vi "Main.vi"(7 "sweep rate, /min":dbl=0.2, 8 "sweep to:":dbl=4.0, 9 "sweep":T8(radio)=enum."2636a_smub") -> ()   [LabVIEW 2021] (continued)
                    }
                    frame True {
                      n3679 = flat-sequence {
                        tunnel: [w4987] -> w4981
                        tunnel: [w4986] -> w4980
                        tunnel: [w4985] -> w4979
                        frame #0 {
                          n3680 = property on="HandleOut" class="Clust (strict)"() -> ("Value"=w4989:T1)  [unwired: 2 in, 2 out]
                          n3681 = call "MFLIcontrol.vi"("MFLI function"=MFLIcommand."measure XY on demod2", "handle in"=w4989) -> ("Demod Sample Out 2"=w4984:T20)  [unwired: 5 in, 4 out]
                          n3682 = Unbundle(w4984) -> ("X (Vrms)"=w4987:dbl, "Y (Vrms)"=w4986:dbl, "Freq (Hz)"=w4985:dbl)  [unwired: 6 out]
                        }
                      }
                      n3683 = Build Array (concatenate)(w4983, w4981, w4980, w4979) -> (w4982:dbl[])
                    }
                  }
                  n3684 = property on="data" class="Arr (strict)"("Value"=w4976) -> ()  [unwired: 2 in, 2 out]
                }
                frame #42 {
                  # "Measure MFLI_V if \nit is checked"
                  n3685 = property on="MFLI1_d3" class="Bool (strict)"() -> ("Value"=w4990:bool)  [unwired: 2 in, 2 out]
                  n3686 = property on="data" class="Arr (strict)"() -> ("Value"=w4992:dbl[])  [unwired: 2 in, 2 out]
                  n3687 = case shown="True" w4990 {
                    tunnel: w4992 -> [w4993 w4998]
                    tunnel: [w4993 w4997] -> w4991
                    frame False {
                      # "We are not recording Step Value if it is linetrace"
                    }
                    frame True {
                      n3688 = flat-sequence {
                        tunnel: [w5002] -> w4996
                        tunnel: [w5001] -> w4995
                        tunnel: [w5000] -> w4994
                        frame #0 {
                          n3689 = property on="HandleOut" class="Clust (strict)"() -> ("Value"=w5004:T1)  [unwired: 2 in, 2 out]
                          n3690 = call "MFLIcontrol.vi"("MFLI function"=MFLIcommand."measure XY on demod3", "handle in"=w5004) -> ("Demod Sample Out 2"=w4999:T20)  [unwired: 5 in, 4 out]
                          n3691 = Unbundle(w4999) -> ("X (Vrms)"=w5002:dbl, "Y (Vrms)"=w5001:dbl, "Freq (Hz)"=w5000:dbl)  [unwired: 6 out]
                        }
                      }
                      n3692 = Build Array (concatenate)(w4998, w4996, w4995, w4994) -> (w4997:dbl[])
                    }
                  }
                  n3693 = property on="data" class="Arr (strict)"("Value"=w4991) -> ()  [unwired: 2 in, 2 out]
                }
                frame #43 {
                  # "Measure MFLI_V if \nit is checked"
                  n3694 = property on="MFLI2_d0" class="Bool (strict)"() -> ("Value"=w5005:bool)  [unwired: 2 in, 2 out]
                  n3695 = property on="data" class="Arr (strict)"() -> ("Value"=w5007:dbl[])  [unwired: 2 in, 2 out]
                  n3696 = case shown="True" w5005 {
                    tunnel: w5007 -> [w5008 w5013]
                    tunnel: [w5008 w5012] -> w5006
                    frame False {
                      # "We are not recording Step Value if it is linetrace"
                    }
                    frame True {
                      n3697 = flat-sequence {
                        tunnel: [w5017] -> w5011
                        tunnel: [w5016] -> w5010
                        tunnel: [w5015] -> w5009
                        frame #0 {
                          n3698 = property on="HandleOut 2" class="Clust (strict)"() -> ("Value"=w5019:T21)  [unwired: 2 in, 2 out]
                          n3699 = call "MFLIcontrol.vi"("MFLI function"=MFLIcommand."measure XY on demod0", "handle in"=w5019) -> ("Demod Sample Out 2"=w5014:T20)  [unwired: 5 in, 4 out]
                          n3700 = Unbundle(w5014) -> ("X (Vrms)"=w5017:dbl, "Y (Vrms)"=w5016:dbl, "Freq (Hz)"=w5015:dbl)  [unwired: 6 out]
                        }
                      }
                      n3701 = Build Array (concatenate)(w5013, w5011, w5010, w5009) -> (w5012:dbl[])
                    }
                  }
                  n3702 = property on="data" class="Arr (strict)"("Value"=w5006) -> ()  [unwired: 2 in, 2 out]
                }
                frame #44 {
                  # "Measure MFLI_V if \nit is checked"
                  n3703 = property on="MFLI2_d1" class="Bool (strict)"() -> ("Value"=w5020:bool)  [unwired: 2 in, 2 out]
                  n3704 = property on="data" class="Arr (strict)"() -> ("Value"=w5022:dbl[])  [unwired: 2 in, 2 out]
                  n3705 = case shown="True" w5020 {
                    tunnel: w5022 -> [w5023 w5028]
                    tunnel: [w5023 w5027] -> w5021
                    frame False {
                      # "We are not recording Step Value if it is linetrace"
                    }
                    frame True {
                      n3706 = flat-sequence {
                        tunnel: [w5032] -> w5026
                        tunnel: [w5031] -> w5025
                        tunnel: [w5030] -> w5024
                        frame #0 {
                          n3707 = property on="HandleOut 2" class="Clust (strict)"() -> ("Value"=w5034:T21)  [unwired: 2 in, 2 out]
                          n3708 = call "MFLIcontrol.vi"("MFLI function"=MFLIcommand."measure XY on demod1", "handle in"=w5034) -> ("Demod Sample Out 2"=w5029:T20)  [unwired: 5 in, 4 out]
                          n3709 = Unbundle(w5029) -> ("X (Vrms)"=w5032:dbl, "Y (Vrms)"=w5031:dbl, "Freq (Hz)"=w5030:dbl)  [unwired: 6 out]
                        }
                      }
                      n3710 = Build Array (concatenate)(w5028, w5026, w5025, w5024) -> (w5027:dbl[])
                    }
                  }
                  n3711 = property on="data" class="Arr (strict)"("Value"=w5021) -> ()  [unwired: 2 in, 2 out]
                }
                frame #45 {
                  # "Measure MFLI_V if \nit is checked"
                  n3712 = property on="MFLI2_d2" class="Bool (strict)"() -> ("Value"=w5035:bool)  [unwired: 2 in, 2 out]
                  n3713 = property on="data" class="Arr (strict)"() -> ("Value"=w5037:dbl[])  [unwired: 2 in, 2 out]
                  n3714 = case shown="True" w5035 {
                    tunnel: w5037 -> [w5038 w5043]
                    tunnel: [w5038 w5042] -> w5036
                    frame False {
                      # "We are not recording Step Value if it is linetrace"
                    }
                    frame True {
                      n3715 = flat-sequence {
                        tunnel: [w5047] -> w5041
                        tunnel: [w5046] -> w5040
                        tunnel: [w5045] -> w5039
                        frame #0 {
                          n3716 = property on="HandleOut 2" class="Clust (strict)"() -> ("Value"=w5049:T21)  [unwired: 2 in, 2 out]
                          n3717 = call "MFLIcontrol.vi"("MFLI function"=MFLIcommand."measure XY on demod2", "handle in"=w5049) -> ("Demod Sample Out 2"=w5044:T20)  [unwired: 5 in, 4 out]
                          n3718 = Unbundle(w5044) -> ("X (Vrms)"=w5047:dbl, "Y (Vrms)"=w5046:dbl, "Freq (Hz)"=w5045:dbl)  [unwired: 6 out]
                        }
                      }
                      n3719 = Build Array (concatenate)(w5043, w5041, w5040, w5039) -> (w5042:dbl[])
                    }
                  }
                  n3720 = property on="data" class="Arr (strict)"("Value"=w5036) -> ()  [unwired: 2 in, 2 out]
                }
                frame #46 {
                  # "Measure MFLI_V if \nit is checked"
                  n3721 = property on="MFLI2_d3" class="Bool (strict)"() -> ("Value"=w5050:bool)  [unwired: 2 in, 2 out]
                  n3722 = property on="data" class="Arr (strict)"() -> ("Value"=w5052:dbl[])  [unwired: 2 in, 2 out]
                  n3723 = case shown="True" w5050 {
                    tunnel: w5052 -> [w5053 w5058]
                    tunnel: [w5053 w5057] -> w5051
                    frame False {
                      # "We are not recording Step Value if it is linetrace"
                    }
                    frame True {
                      n3724 = flat-sequence {
                        tunnel: [w5062] -> w5056
                        tunnel: [w5061] -> w5055
                        tunnel: [w5060] -> w5054
                        frame #0 {
                          n3725 = property on="HandleOut 2" class="Clust (strict)"() -> ("Value"=w5064:T21)  [unwired: 2 in, 2 out]
                          n3726 = call "MFLIcontrol.vi"("MFLI function"=MFLIcommand."measure XY on demod3", "handle in"=w5064) -> ("Demod Sample Out 2"=w5059:T20)  [unwired: 5 in, 4 out]
                          n3727 = Unbundle(w5059) -> ("X (Vrms)"=w5062:dbl, "Y (Vrms)"=w5061:dbl, "Freq (Hz)"=w5060:dbl)  [unwired: 6 out]
                        }
                      }
                      n3728 = Build Array (concatenate)(w5058, w5056, w5055, w5054) -> (w5057:dbl[])
                    }
                  }
                  n3729 = property on="data" class="Arr (strict)"("Value"=w5051) -> ()  [unwired: 2 in, 2 out]
                }
                frame #47 {
                  # "Measure MFLI_V if \nit is checked"
                  n3730 = property on="MFLI3_d0" class="Bool (strict)"() -> ("Value"=w5065:bool)  [unwired: 2 in, 2 out]
                  n3731 = property on="data" class="Arr (strict)"() -> ("Value"=w5067:dbl[])  [unwired: 2 in, 2 out]
                  n3732 = case shown="True" w5065 {
                    tunnel: w5067 -> [w5068 w5073]
                    tunnel: [w5068 w5072] -> w5066
                    frame False {
                      # "We are not recording Step Value if it is linetrace"
                    }
                    frame True {
                      n3733 = flat-sequence {
                        tunnel: [w5077] -> w5071
                        tunnel: [w5076] -> w5070
                        tunnel: [w5075] -> w5069
                        frame #0 {
                          n3734 = property on="HandleOut 3" class="Clust (strict)"() -> ("Value"=w5079:T1)  [unwired: 2 in, 2 out]
                          n3735 = call "MFLIcontrol.vi"("MFLI function"=MFLIcommand."measure XY on demod0", "handle in"=w5079) -> ("Demod Sample Out 2"=w5074:T20)  [unwired: 5 in, 4 out]
                          n3736 = Unbundle(w5074) -> ("X (Vrms)"=w5077:dbl, "Y (Vrms)"=w5076:dbl, "Freq (Hz)"=w5075:dbl)  [unwired: 6 out]
                        }
                      }
                      n3737 = Build Array (concatenate)(w5073, w5071, w5070, w5069) -> (w5072:dbl[])
                    }
                  }
                  n3738 = property on="data" class="Arr (strict)"("Value"=w5066) -> ()  [unwired: 2 in, 2 out]
                }
                frame #48 {
                  # "Measure MFLI_V if \nit is checked"
                  n3739 = property on="MFLI3_d1" class="Bool (strict)"() -> ("Value"=w5080:bool)  [unwired: 2 in, 2 out]
                  n3740 = property on="data" class="Arr (strict)"() -> ("Value"=w5082:dbl[])  [unwired: 2 in, 2 out]
                  n3741 = case shown="True" w5080 {
                    tunnel: w5082 -> [w5083 w5088]
                    tunnel: [w5083 w5087] -> w5081
                    frame False {
                      # "We are not recording Step Value if it is linetrace"
                    }
                    frame True {
                      n3742 = flat-sequence {
                        tunnel: [w5092] -> w5086
                        tunnel: [w5091] -> w5085
                        tunnel: [w5090] -> w5084
                        frame #0 {
                          n3743 = property on="HandleOut 3" class="Clust (strict)"() -> ("Value"=w5094:T1)  [unwired: 2 in, 2 out]
                          n3744 = call "MFLIcontrol.vi"("MFLI function"=MFLIcommand."measure XY on demod1", "handle in"=w5094) -> ("Demod Sample Out 2"=w5089:T20)  [unwired: 5 in, 4 out]
                          n3745 = Unbundle(w5089) -> ("X (Vrms)"=w5092:dbl, "Y (Vrms)"=w5091:dbl, "Freq (Hz)"=w5090:dbl)  [unwired: 6 out]
                        }
                      }
                      n3746 = Build Array (concatenate)(w5088, w5086, w5085, w5084) -> (w5087:dbl[])
                    }
                  }
                  n3747 = property on="data" class="Arr (strict)"("Value"=w5081) -> ()  [unwired: 2 in, 2 out]
                }
                frame #49 {
                  # "Measure MFLI_V if \nit is checked"
                  n3748 = property on="MFLI3_d2" class="Bool (strict)"() -> ("Value"=w5095:bool)  [unwired: 2 in, 2 out]
                  n3749 = property on="data" class="Arr (strict)"() -> ("Value"=w5097:dbl[])  [unwired: 2 in, 2 out]
                  n3750 = case shown="True" w5095 {
                    tunnel: w5097 -> [w5098 w5103]
                    tunnel: [w5098 w5102] -> w5096
                    frame False {
                      # "We are not recording Step Value if it is linetrace"
                    }
                    frame True {
                      n3751 = flat-sequence {
                        tunnel: [w5107] -> w5101
                        tunnel: [w5106] -> w5100
                        tunnel: [w5105] -> w5099
                        frame #0 {
                          n3752 = property on="HandleOut 3" class="Clust (strict)"() -> ("Value"=w5109:T1)  [unwired: 2 in, 2 out]
                          n3753 = call "MFLIcontrol.vi"("MFLI function"=MFLIcommand."measure XY on demod2", "handle in"=w5109) -> ("Demod Sample Out 2"=w5104:T20)  [unwired: 5 in, 4 out]
                          n3754 = Unbundle(w5104) -> ("X (Vrms)"=w5107:dbl, "Y (Vrms)"=w5106:dbl, "Freq (Hz)"=w5105:dbl)  [unwired: 6 out]
                        }
                      }
                      n3755 = Build Array (concatenate)(w5103, w5101, w5100, w5099) -> (w5102:dbl[])
                    }
                  }
                  n3756 = property on="data" class="Arr (strict)"("Value"=w5096) -> ()  [unwired: 2 in, 2 out]
                }
                frame #50 {
                  # "Measure MFLI_V if \nit is checked"
                  n3757 = property on="MFLI3_d3" class="Bool (strict)"() -> ("Value"=w5110:bool)  [unwired: 2 in, 2 out]
                  n3758 = property on="data" class="Arr (strict)"() -> ("Value"=w5112:dbl[])  [unwired: 2 in, 2 out]
                  n3759 = case shown="True" w5110 {
                    tunnel: w5112 -> [w5113 w5118]
                    tunnel: [w5113 w5117] -> w5111
                    frame False {
                      # "We are not recording Step Value if it is linetrace"
                    }
                    frame True {
                      n3760 = flat-sequence {
                        tunnel: [w5122] -> w5116
                        tunnel: [w5121] -> w5115
                        tunnel: [w5120] -> w5114
                        frame #0 {
                          n3761 = property on="HandleOut 3" class="Clust (strict)"() -> ("Value"=w5124:T1)  [unwired: 2 in, 2 out]
                          n3762 = call "MFLIcontrol.vi"("MFLI function"=MFLIcommand."measure XY on demod3", "handle in"=w5124) -> ("Demod Sample Out 2"=w5119:T20)  [unwired: 5 in, 4 out]
                          n3763 = Unbundle(w5119) -> ("X (Vrms)"=w5122:dbl, "Y (Vrms)"=w5121:dbl, "Freq (Hz)"=w5120:dbl)  [unwired: 6 out]
                        }
                      }
                      n3764 = Build Array (concatenate)(w5118, w5116, w5115, w5114) -> (w5117:dbl[])
                    }
                  }
                  n3765 = property on="data" class="Arr (strict)"("Value"=w5111) -> ()  [unwired: 2 in, 2 out]
                }
                frame #51 {
                  # "Measure MFLI_V if \nit is checked"
                  n3766 = property on="MFLI4_d0" class="Bool (strict)"() -> ("Value"=w5125:bool)  [unwired: 2 in, 2 out]
                  n3767 = property on="data" class="Arr (strict)"() -> ("Value"=w5127:dbl[])  [unwired: 2 in, 2 out]
                  n3768 = case shown="True" w5125 {
                    tunnel: w5127 -> [w5128 w5133]
                    tunnel: [w5128 w5132] -> w5126
                    frame False {
                      # "We are not recording Step Value if it is linetrace"
                    }
                    frame True {
                      n3769 = flat-sequence {
                        tunnel: [w5137] -> w5131
                        tunnel: [w5136] -> w5130
                        tunnel: [w5135] -> w5129
                        frame #0 {
                          n3770 = property on="HandleOut 4" class="Clust (strict)"() -> ("Value"=w5139:T21)  [unwired: 2 in, 2 out]
                          n3771 = call "MFLIcontrol.vi"("MFLI function"=MFLIcommand."measure XY on demod0", "handle in"=w5139) -> ("Demod Sample Out 2"=w5134:T20)  [unwired: 5 in, 4 out]
                          n3772 = Unbundle(w5134) -> ("X (Vrms)"=w5137:dbl, "Y (Vrms)"=w5136:dbl, "Freq (Hz)"=w5135:dbl)  [unwired: 6 out]
                        }
                      }
                      n3773 = Build Array (concatenate)(w5133, w5131, w5130, w5129) -> (w5132:dbl[])
                    }
                  }
                  n3774 = property on="data" class="Arr (strict)"("Value"=w5126) -> ()  [unwired: 2 in, 2 out]
                }
                frame #52 {
                  # "Measure MFLI_V if \nit is checked"
                  n3775 = property on="MFLI4_d1" class="Bool (strict)"() -> ("Value"=w5140:bool)  [unwired: 2 in, 2 out]
                  n3776 = property on="data" class="Arr (strict)"() -> ("Value"=w5142:dbl[])  [unwired: 2 in, 2 out]
                  n3777 = case shown="True" w5140 {
                    tunnel: w5142 -> [w5143 w5148]
                    tunnel: [w5143 w5147] -> w5141
                    frame False {
                      # "We are not recording Step Value if it is linetrace"
                    }
                    frame True {
                      n3778 = flat-sequence {
                        tunnel: [w5152] -> w5146
                        tunnel: [w5151] -> w5145
                        tunnel: [w5150] -> w5144
                        frame #0 {
                          n3779 = property on="HandleOut 4" class="Clust (strict)"() -> ("Value"=w5154:T21)  [unwired: 2 in, 2 out]
                          n3780 = call "MFLIcontrol.vi"("MFLI function"=MFLIcommand."measure XY on demod1", "handle in"=w5154) -> ("Demod Sample Out 2"=w5149:T20)  [unwired: 5 in, 4 out]
                          n3781 = Unbundle(w5149) -> ("X (Vrms)"=w5152:dbl, "Y (Vrms)"=w5151:dbl, "Freq (Hz)"=w5150:dbl)  [unwired: 6 out]
                        }
                      }
                      n3782 = Build Array (concatenate)(w5148, w5146, w5145, w5144) -> (w5147:dbl[])
                    }
                  }
                  n3783 = property on="data" class="Arr (strict)"("Value"=w5141) -> ()  [unwired: 2 in, 2 out]
                }
                frame #53 {
                  # "Measure MFLI_V if \nit is checked"
                  n3784 = property on="MFLI4_d2" class="Bool (strict)"() -> ("Value"=w5155:bool)  [unwired: 2 in, 2 out]
                  n3785 = property on="data" class="Arr (strict)"() -> ("Value"=w5157:dbl[])  [unwired: 2 in, 2 out]
                  n3786 = case shown="True" w5155 {
                    tunnel: w5157 -> [w5158 w5163]
                    tunnel: [w5158 w5162] -> w5156
                    frame False {
                      # "We are not recording Step Value if it is linetrace"
                    }
                    frame True {
                      n3787 = flat-sequence {
                        tunnel: [w5167] -> w5161
                        tunnel: [w5166] -> w5160
                        tunnel: [w5165] -> w5159
                        frame #0 {
                          n3788 = property on="HandleOut 4" class="Clust (strict)"() -> ("Value"=w5169:T21)  [unwired: 2 in, 2 out]
                          n3789 = call "MFLIcontrol.vi"("MFLI function"=MFLIcommand."measure XY on demod2", "handle in"=w5169) -> ("Demod Sample Out 2"=w5164:T20)  [unwired: 5 in, 4 out]
                          n3790 = Unbundle(w5164) -> ("X (Vrms)"=w5167:dbl, "Y (Vrms)"=w5166:dbl, "Freq (Hz)"=w5165:dbl)  [unwired: 6 out]
                        }
                      }
                      n3791 = Build Array (concatenate)(w5163, w5161, w5160, w5159) -> (w5162:dbl[])
                    }
                  }
                  n3792 = property on="data" class="Arr (strict)"("Value"=w5156) -> ()  [unwired: 2 in, 2 out]
                }
                frame #54 {
                  # "Measure MFLI_V if \nit is checked"
                  n3793 = property on="MFLI4_d3" class="Bool (strict)"() -> ("Value"=w5170:bool)  [unwired: 2 in, 2 out]
                  n3794 = property on="data" class="Arr (strict)"() -> ("Value"=w5172:dbl[])  [unwired: 2 in, 2 out]
                  n3795 = case shown="True" w5170 {
                    tunnel: w5172 -> [w5173 w5178]
                    tunnel: [w5173 w5177] -> w5171
                    frame False {
                      # "We are not recording Step Value if it is linetrace"
                    }
                    frame True {
                      n3796 = flat-sequence {
                        tunnel: [w5182] -> w5176
                        tunnel: [w5181] -> w5175
                        tunnel: [w5180] -> w5174
                        frame #0 {
                          n3797 = property on="HandleOut 4" class="Clust (strict)"() -> ("Value"=w5184:T21)  [unwired: 2 in, 2 out]
                          n3798 = call "MFLIcontrol.vi"("MFLI function"=MFLIcommand."measure XY on demod3", "handle in"=w5184) -> ("Demod Sample Out 2"=w5179:T20)  [unwired: 5 in, 4 out]
                          n3799 = Unbundle(w5179) -> ("X (Vrms)"=w5182:dbl, "Y (Vrms)"=w5181:dbl, "Freq (Hz)"=w5180:dbl)  [unwired: 6 out]
                        }
                      }
                      n3800 = Build Array (concatenate)(w5178, w5176, w5175, w5174) -> (w5177:dbl[])
                    }
                  }
                  n3801 = property on="data" class="Arr (strict)"("Value"=w5171) -> ()  [unwired: 2 in, 2 out]
                }
                frame #55 {
                  # "Measure MFLI_V if \nit is checked"
                  n3802 = property on="MFLI1_AuxOut0" class="Bool (strict)"() -> ("Value"=w5185:bool)  [unwired: 2 in, 2 out]
                  n3803 = property on="data" class="Arr (strict)"() -> ("Value"=w5187:dbl[])  [unwired: 2 in, 2 out]
                  n3804 = case shown="True" w5185 {
                    tunnel: w5187 -> [w5188 w5190]
                    tunnel: [w5188 w5191] -> w5186
                    frame False {
                      # "We are not recording Step Value if it is linetrace"
                    }
                    frame True {
                      n3805 = flat-sequence {
                        tunnel: [w5192] -> w5189
                        frame #0 {
                          n3806 = property on="HandleOut" class="Clust (strict)"() -> ("Value"=w5194:T1)  [unwired: 2 in, 2 out]
                          n3807 = call "MFLIcontrol.vi"("MFLI function"=MFLIcommand."Get AuxOut0", "handle in"=w5194) -> ("AuxOut0_Ampl"=w5192:dbl)  [unwired: 5 in, 4 out]
                        }
                      }
                      n3808 = Build Array (concatenate)(w5190, w5189) -> (w5191:dbl[])
                    }
                  }
                  n3809 = property on="data" class="Arr (strict)"("Value"=w5186) -> ()  [unwired: 2 in, 2 out]
                }
              }
            }
            frame #4 {
              n3810 = property on="data" class="Arr (strict)"() -> ("Value"=w5195:dbl[])  [unwired: 2 in, 2 out]
            }
          }
          n3811 = stacked-sequence "add data to array" {
            tunnel: w4336 -> [w4348]
            tunnel: [w4347] -> w4335
            tunnel: w4334 -> [w4346]
            frame #0 {
              n3812 = Build Array (concatenate)(w4348, w4346) -> (w4347:dbl[][])
            }
          }
          n3813 = stacked-sequence "plot selected measurements" {
            seq-local: [_ w4371 _] -> [_ _ w4416]
            seq-local: [_ w4370 _] -> [_ _ w4417]
            tunnel: w4335 -> [_ w4369 _]
            frame #0 {
              n3814 = property on="XY Graph" class="XYGraph (strict)"("ActYScl"=0 ("Active Y Scale")) -> (error out=w4354:errorcluster)  [unwired: 2 in, 1 out]
              n3815 = property on="Show cursor" class="Bool (strict)"() -> ("Value"=w4349:bool)  [unwired: 2 in, 2 out]
              n3816 = property on="Xaxis" class="Ring (strict)"() -> ("Value"=w4359:u16)  [unwired: 2 in, 2 out]
              n3817 = property on="Yaxis" class="Ring (strict)"(error in=w4354) -> (error out=w4353:errorcluster, "RingText.Text"=w4352:string)  [unwired: 1 in, 1 out]
              n3818 = property on="XY Graph" class="XYGraph (strict)"("Cursor.Visible"=w4349) -> ()  [unwired: 2 in, 2 out]
              n3819 = property on="Figure_axis" class="Arr (strict)"() -> ("Value"=w4360:string[])  [unwired: 2 in, 2 out]
              n3820 = property on="XY Graph" class="XYGraph (strict)"(error in=w4353, "YScale.NameLbl.Text"=w4352) -> (error out=w4350:errorcluster)  [unwired: 1 in, 1 out]
              n3821 = property on="XY Graph" class="XYGraph (strict)"(error in=w4350, "ActYScl"=1 ("Active Y Scale")) -> (error out=w4356:errorcluster)  [unwired: 1 in, 1 out]
              n3822 = property on="Yright" class="Ring (strict)"(error in=w4356) -> (error out=w4357:errorcluster, "RingText.Text"=w4351:string)  [unwired: 1 in, 1 out]
              n3823 = Index Array(array=w4360, index=w4359) -> (element=w4361:string)
              n3824 = property on="XY Graph" class="XYGraph (strict)"("XScale.NameLbl.Text"=w4361) -> ()  [unwired: 2 in, 2 out]
              n3825 = property on="XY Graph" class="XYGraph (strict)"(error in=w4357, "YScale.NameLbl.Text"=w4351) -> ()  [unwired: 1 in, 2 out]
            }
            frame #1 {
              n3826 = local read "Xaxis"() -> (w4374:u16)
              n3827 = property on="Yright" class="Ring (strict)"() -> ("Value"=w4368:u16)  [unwired: 2 in, 2 out]
              n3828 = property on="Yright" class="Ring (strict)"() -> ("RingText.Text"=w4367:string)  [unwired: 2 in, 2 out]
              n3829 = property on="Xaxis" class="Ring (strict)"() -> ("RingText.Text"=w4373:string)  [unwired: 2 in, 2 out]
              n3830 = property on="Yaxis" class="Ring (strict)"() -> ("RingText.Text"=w4372:string)  [unwired: 2 in, 2 out]
              n3831 = local read "Yaxis"() -> (w4375:u16)
              n3832 = case shown="\"formula\"" w4367 {
                tunnel: [w4380 w4387] -> w4365
                tunnel: w4368 -> [_ w4386]
                tunnel: w4369 -> [w4381 w4385]
                tunnel: [w4379 errorcluster {"status"=FALSE, "code"=0, "source"=""} ("error out")] -> _
                frame "formula" {
                  n3833 = local read "formula_variables"() -> (w4382:string[])
                  n3834 = Transpose 2D Array(2D array=w4381) -> (transposed array=w4383:dbl[][])
                  n3835 = property on="Y_right_formula" class="Str"() -> ("Value"=w4378:string)  [unwired: 2 in, 2 out]
                  n3836 = call <vilib>:"Eval Multi-Variable Array.vi"("Variables"=w4382, "X Values"=w4383, "formula"=w4378) -> ("error out"=w4379:errorcluster, "Y Values"=w4380:dbl[])  [unwired: 1 in]
                }
                frame "0", Default {
                  n3837 = Index Array(array=w4385, index (col)=w4386) -> (element=w4387:dbl[])  [unwired: 1 in]
                }
              }
              n3838 = case shown="\"formula\"" w4373 {
                tunnel: [w4398 w4403] -> w4377
                tunnel: w4374 -> [w4401 _]
                tunnel: w4369 -> [w4400 w4407]
                tunnel: [errorcluster {"status"=FALSE, "code"=0, "source"=""} ("error out") w4404] -> w4371
                tunnel: [w4398 w4403] -> w4366
                frame "0", Default {
                  n3839 = Index Array(array=w4400, index (col)=w4401) -> (element=w4398:dbl[])  [unwired: 1 in]
                }
                frame "formula" {
                  n3840 = local read "formula_variables"() -> (w4406:string[])
                  n3841 = Transpose 2D Array(2D array=w4407) -> (transposed array=w4405:dbl[][])
                  n3842 = property on="X_axis_formula" class="Str"() -> ("Value"=w4402:string)  [unwired: 2 in, 2 out]
                  n3843 = call <vilib>:"Eval Multi-Variable Array.vi"("Variables"=w4406, "X Values"=w4405, "formula"=w4402) -> ("error out"=w4404:errorcluster, "Y Values"=w4403:dbl[])  [unwired: 1 in]
                }
              }
              n3844 = case shown="\"formula\"" w4372 {
                tunnel: [w4390 w4397] -> w4376
                tunnel: w4375 -> [_ w4396]
                tunnel: w4369 -> [w4391 w4395]
                tunnel: [w4389 errorcluster {"status"=FALSE, "code"=0, "source"=""} ("error out")] -> w4370
                frame "formula" {
                  n3845 = local read "formula_variables"() -> (w4392:string[])
                  n3846 = Transpose 2D Array(2D array=w4391) -> (transposed array=w4393:dbl[][])
                  n3847 = property on="Y_left_formula" class="Str"() -> ("Value"=w4388:string)  [unwired: 2 in, 2 out]
                  n3848 = call <vilib>:"Eval Multi-Variable Array.vi"("Variables"=w4392, "X Values"=w4393, "formula"=w4388) -> ("error out"=w4389:errorcluster, "Y Values"=w4390:dbl[])  [unwired: 1 in]
                }
                frame "0", Default {
                  n3849 = Index Array(array=w4395, index (col)=w4396) -> (element=w4397:dbl[])  [unwired: 1 in]
                }
              }
              n3850 = Bundle("Y Values"=w4377, "Y Values"=w4376) -> (w4364:cluster{"Y Values":dbl[], "Y Values":dbl[]})  [unwired: 1 in]
              n3851 = Bundle("Y Values"=w4366, "Y Values"=w4365) -> (w4363:cluster{"Y Values":dbl[], "Y Values":dbl[]})  [unwired: 1 in]
              n3852 = Build Array(w4364, w4363) -> (w4362:cluster{"Y Values":dbl[], "Y Values":dbl[]}[])
              n3853 = property on="XY Graph" class="XYGraph (strict)"("Value"=w4362) -> ()  [unwired: 2 in, 2 out]
            }
            frame #2 {
              # "show if formula \nis wrong"
              n3854 = property on="Yaxis" class="Ring (strict)"() -> ("RingText.Text"=w4413:string)  [unwired: 2 in, 2 out]
              n3855 = property on="XY Graph" class="XYGraph (strict)"("Active Plot"=u32 0, "Plot.Plot Name"=w4413) -> (error out=w4414:errorcluster)  [unwired: 2 in, 1 out]
              n3856 = property on="Yright" class="Ring (strict)"() -> ("RingText.Text"=w4411:string)  [unwired: 2 in, 2 out]
              n3857 = property on="XY Graph" class="XYGraph (strict)"(error in=w4414, "Active Plot"=u32 1, "Plot.Plot Name"=w4411) -> ()  [unwired: 1 in, 2 out]
              n3858 = Unbundle By Name(w4417) -> ("status"=w4410:bool)
              n3859 = Unbundle By Name(w4416) -> ("status"=w4409:bool)
              n3860 = Unbundle By Name(w4416) -> ("status"=w4408:bool)
              n3861 = property on="status 3" class="Bool (strict)"("Value"=w4408) -> ()  [unwired: 2 in, 2 out]
              n3862 = property on="status 2" class="Bool (strict)"("Value"=w4410) -> ()  [unwired: 2 in, 2 out]
              n3863 = property on="status" class="Bool (strict)"("Value"=w4409) -> ()  [unwired: 2 in, 2 out]
            }
          }
          n3864 = stacked-sequence "set next value in the sweep" {
            tunnel: w4345 -> [w5201 _]
            tunnel: [w5201 _] -> w4344
            tunnel: w4342 -> [_ w5317]
            tunnel: w4340 -> [w5204 _]
            frame #0 {
              n3865 = local read "sweep"() -> (w5207:T8)
              n3866 = property on="Sweep Channel" class="DigNum (strict)"("Value"=w5201) -> ()  [unwired: 2 in, 2 out]
              n3867 = property on="sweep value" class="DigNum (strict)"("Value"=w5201) -> ()  [unwired: 2 in, 2 out]
              n3868 = case shown="\"AuxOut0\"" w5207 {
                tunnel: w5201 -> [w5220 w5228 w5234 w5243 w5265 _ w5267 w5290 w5308 w5311]
                tunnel: w5204 -> [_ _ _ w5242 _ _ _ _ _ _]
                frame "2400_1" {
                  # "sweep voltage on 2400 1"
                  n3869 = local read "2400 1 addr"() -> (w5222:u8)
                  n3870 = Number To Fractional String(number=w5220) -> (F-format string=w5226:string)  [unwired: 3 in]
                  n3871 = Concatenate Strings(":INIT:IMM; :SOUR:VOLT:LEV:IMM:AMPL " ("data"), w5226) -> (w5224:string)
                  n3872 = Number To Decimal String(number=w5222) -> (decimal integer string=w5221:string)  [unwired: 1 in]
                  n3873 = GPIB Write(0:w5221, 1:w5224, 2:i16 1 ("mode (0)")) -> ()  [unwired: 2 in, 2 out]
                }
                frame "2400_2" {
                  # "sweep curr on 2400 2"
                  n3874 = Number To Fractional String(number=w5228) -> (F-format string=w5233:string)  [unwired: 3 in]
                  n3875 = local read "2400 2 addr"() -> (w5230:u8)
                  n3876 = Concatenate Strings(":INIT:IMM; :SOUR:CURR:LEV:IMM:AMPL " ("data"), w5233) -> (w5231:string)
                  n3877 = Number To Decimal String(number=w5230) -> (decimal integer string=w5229:string)  [unwired: 1 in]
                  n3878 = GPIB Write(0:w5229, 1:w5231, 2:i16 1 ("mode (0)")) -> ()  [unwired: 2 in, 2 out]
                }
                frame "2400_3" {
                  # "sweep voltage on 2400 3"
                  n3879 = local read "2400 3 addr"() -> (w5236:u8)
                  n3880 = Number To Fractional String(number=w5234) -> (F-format string=w5240:string)  [unwired: 3 in]
                  n3881 = Concatenate Strings(":INIT:IMM; :SOUR:VOLT:LEV:IMM:AMPL " ("data"), w5240) -> (w5238:string)
                  n3882 = Number To Decimal String(number=w5236) -> (decimal integer string=w5235:string)  [unwired: 1 in]
                  n3883 = GPIB Write(0:w5235, 1:w5238, 2:i16 1 ("mode (0)")) -> ()  [unwired: 2 in, 2 out]
                }
                frame "2636a_smua" {
                  n3884 = property on="sweep" class="Bool (strict)"() -> ("Value"=w5241:bool)  [unwired: 2 in, 2 out]
                  n3885 = case shown="False" w5241 {
                    tunnel: w5243 -> [w5248 w5261]
                    tunnel: w5242 -> [w5245 _]
                    frame True {
                      w5246 = 30.0 ("y")
                      n3886 = Subtract(x=w5248, y=w5245) -> (x-y=w5247:dbl)
                      n3887 = Divide(x=w5247, y=w5246) -> (x/y=w5244:dbl)
                      n3888 = for {
                        N: w5246 -> [_]
                        tunnel: w5245 -> [w5254]
                        tunnel: w5244 -> [w5252]
                        i -> [w5253]
                        n3889 = Multiply(x=w5252, y=w5253) -> (x*y=w5251:dbl)
                        n3890 = local read "2614A addr"() -> (w5256:refnum<visa-resource-name>)
                        n3891 = Add(x=w5251, y=w5254) -> (x+y=w5250:dbl)
                        n3892 = call "setLevel.vi"("VISA resource name 2"=w5256, "Source"=Source."Voltage", "Channel"=Channel."a", "SourceLevel"=w5250) -> ()  [unwired: 1 in, 3 out]
                        n3893 = Wait (ms)(milliseconds to wait=u32 12) -> ()  [unwired: 1 out]
                      }
                    }
                    frame False {
                      # "sweep voltage on 2636a smua"
                      n3894 = local read "2614A addr"() -> (w5259:refnum<visa-resource-name>)
                      n3895 = call "setLevel.vi"("VISA resource name 2"=w5259, "Source"=Source."Voltage", "Channel"=Channel."a", "SourceLevel"=w5261) -> ()  [unwired: 1 in, 3 out]
                    }
                  }
                }
                frame "2636a_smub" {
                  # "sweep voltage on 2636b smua"
                  n3896 = local read "2614A addr"() -> (w5262:refnum<visa-resource-name>)
                  n3897 = call "setLevel.vi"("VISA resource name 2"=w5262, "Source"=Source."Voltage", "Channel"=Channel."b", "SourceLevel"=w5265) -> ()  [unwired: 1 in, 3 out]
                }
                frame "time_sweep", Default {
                  # "do not sweep, just time"
                }
                frame "iPS" {
                  n3898 = property on="Sweep B" class="Bool (strict)"() -> ("Value"=w5266:bool)  [unwired: 2 in, 2 out]
                  n3899 = case shown="True" w5266 {
                    tunnel: w5267 -> [_ w5268]
                    frame False {
                    }
                    frame True {
                      n3900 = stacked-sequence {
                        tunnel: w5268 -> [w5269 _ w5279 w5281]
                        frame #0 {
                          n3901 = local read "iPS_addr_sweep"() -> (w5271:refnum<visa-resource-name>)
                          n3902 = call "iPSset.vi"("Target Field, T"=w5269, "iPSSetCtrl"=iPSsetCtrl."Set Target Field", "VISA resource name"=w5271) -> ()  [unwired: 5 in, 4 out]
                        }
                        frame #1 {
                          n3903 = local read "iPS_addr_sweep"() -> (w5274:refnum<visa-resource-name>)
                          n3904 = call "iPSset.vi"("Field Rate, T/min"=0.15, "iPSSetCtrl"=iPSsetCtrl."Set Target Field Rate", "VISA resource name"=w5274) -> ()  [unwired: 5 in, 4 out]
                        }
                        frame #2 {
                          n3905 = Not Equal To 0?(x=w5279) -> (x != 0?=w5277:bool)
                          n3906 = local read "iPS_addr_sweep"() -> (w5280:refnum<visa-resource-name>)
                          n3907 = Select(t=iPSsetCtrl."Go to Field" ("iPSSetCtrl"), s=w5277, f=iPSsetCtrl."Go to Field" ("iPSSetCtrl")) -> (s? t:f=w5275:T16)
                          n3908 = call "iPSset.vi"("iPSSetCtrl"=w5275, "VISA resource name"=w5280) -> ()  [unwired: 6 in, 4 out]
                        }
                        frame #3 {
                          n3909 = while {
                            tunnel: w5281 -> [w5283]
                            stop <- w5287 stop-if-true
                            n3910 = property on="iPS _addr_step" class="VISAName"() -> ("Value"=w5286:refnum<visa-resource-name>)  [unwired: 2 in, 2 out]
                            n3911 = call "iPSread.vi"("iPSreadCtrl"=iPSreadCtrl."MagnetField", "VISA resource name"=w5286) -> ("number"=w5285:dbl)  [unwired: 6 in, 3 out]
                            n3912 = Subtract(x=w5285, y=w5283) -> (x-y=w5289:dbl)
                            n3913 = property on="Tolerance_Sweep" class="DigNum (strict)"() -> ("Value"=w5284:dbl)  [unwired: 2 in, 2 out]
                            n3914 = Absolute Value(x=w5289) -> (abs(x)=w5288:dbl)
                            n3915 = Less Or Equal?(x=w5288, y=w5284) -> (x <= y?=w5287:bool)
                          }
                        }
                      }
                    }
                  }
                }
                frame "iTC" {
                  n3916 = stacked-sequence {
                    tunnel: w5290 -> [w5292 w5297 w5300]
                    frame #0 {
                      n3917 = Decrement(x=w5292) -> (x-1=w5293:dbl)
                      n3918 = Less Or Equal To 0?(x=w5293) -> (x <= 0?=w5295:bool)
                      n3919 = Select(t=0.0, s=w5295, f=w5293) -> (s? t:f=w5291:dbl)
                      n3920 = call "TRITON_Set Temperature.vi"("setpoint"=w5291) -> ()  [unwired: 2 in, 1 out]
                    }
                    frame #1 {
                      n3921 = Less Or Equal To 0?(x=w5297) -> (x <= 0?=w5299:bool)
                      n3922 = Select(t=0.0, s=w5299, f=w5297) -> (s? t:f=w5296:dbl)
                      n3923 = call "TRITON_Set Temperature.vi"("setpoint"=w5296) -> ()  [unwired: 2 in, 1 out]
                    }
                    frame #2 {
                      n3924 = while {
                        tunnel: w5300 -> [w5304]
                        stop <- w5305 stop-if-true
                        n3925 = call "TRITON_Read Temperature.vi"("Channel"="T_Channel_sweep") -> ("Measuremet"=w5302:dbl)  [unwired: 1 in, 1 out]
                        n3926 = Subtract(x=w5302, y=w5304) -> (x-y=w5307:dbl)
                        n3927 = property on="Tolerance_Sweep" class="DigNum (strict)"() -> ("Value"=w5303:dbl)  [unwired: 2 in, 2 out]
                        n3928 = Absolute Value(x=w5307) -> (abs(x)=w5306:dbl)
                        n3929 = Less?(x=w5306, y=w5303) -> (x < y?=w5305:bool)
                      }
                    }
                  }
                }
                frame "2461" {
                  w5309 = u16 1 items=["Volts", "Current"] ("Function (0: Volts)")
                  n3930 = property on="2461_addr_sweep" class="VISAName"() -> ("Value"=w5310:refnum<visa-resource-name>)  [unwired: 2 in, 2 out]
                  n3931 = call <instrlib>:"Configure Source Level.vi"("Source Level (1.0)"=w5308, "Function (0: Volts)"=w5309, "VISA resource name"=w5310) -> ()  [unwired: 7 in, 2 out]
                }
                frame "AuxOut0" {
                  n3932 = property on="HandleOut" class="Clust (strict)"() -> ("Value"=w5313:T1)  [unwired: 2 in, 2 out]
                  n3933 = call "MFLIcontrol.vi"("Value"=w5311, "MFLI function"=MFLIcommand."Set AuxOut0", "handle in"=w5313) -> ()  [unwired: 4 in, 5 out]
                }
              }
              n3934 = property on="Offset" class="DigNum (strict)"() -> ("Value"=w5203:dbl)  [unwired: 2 in, 2 out]
              n3935 = property on="Slope" class="DigNum (strict)"() -> ("Value"=w5202:dbl)  [unwired: 2 in, 2 out]
              n3936 = Multiply(x=w5202, y=w5201) -> (x*y=w5205:dbl)
              n3937 = local read "sweep"() -> (w5200:T8)
              n3938 = property on="Lead Chanl" class="Enum (strict)"() -> ("Value"=w5199:T2)  [unwired: 2 in, 2 out]
              n3939 = property on="Double Sweep" class="Bool (strict)"() -> ("Value"=w5197:bool)  [unwired: 2 in, 2 out]
              n3940 = Add(x=w5203, y=w5205) -> (x+y=w5206:dbl)
              n3941 = Equal?(x=w5200, y=w5199) -> (x = y?=w5198:bool)
              n3942 = And(x=w5197, y=w5198) -> (x .and. y?=w5196:bool)
              n3943 = case shown="True" w5196 {
                tunnel: w5206 -> [_ w5208]
                frame False {
                }
                frame True {
                  n3944 = disable-structure shown="Enabled" {
                    disable-tunnel: w5208 -> [w5209 w5217]
                    frame Disabled {
                      # "sweep voltage on 2400 2"
                      n3945 = local read "2400 2 addr"() -> (w5210:u8)
                      n3946 = Number To Fractional String(number=w5209) -> (F-format string=w5211:string)  [unwired: 3 in]
                      n3947 = Concatenate Strings(":INIT:IMM; :SOUR:VOLT:LEV:IMM:AMPL " ("data"), w5211) -> (w5213:string)
                      n3948 = Number To Decimal String(number=w5210) -> (decimal integer string=w5214:string)  [unwired: 1 in]
                      n3949 = GPIB Write(0:w5214, 1:w5213, 2:i16 1 ("mode (0)")) -> ()  [unwired: 2 in, 2 out]
                    }
                    frame Enabled {
                      n3950 = property on="Slave Channel" class="Enum (strict)"() -> ("Value"=w5216:T3)  [unwired: 2 in, 2 out]
                      n3951 = local read "2614A addr"() -> (w5219:refnum<visa-resource-name>)
                      n3952 = call "setLevel.vi"("VISA resource name 2"=w5219, "Source"=Source."Voltage", "Channel"=w5216, "SourceLevel"=w5217) -> ()  [unwired: 1 in, 3 out]
                    }
                  }
                }
              }
            }
            frame #1 {
              # "calculate deliberate time delay for the next step"
              n3953 = Tick Count (ms)() -> (millisecond timer value=w5319:u32)
              n3954 = Subtract(x=w5319, y=w5317) -> (x-y=w5318:u32)
              n3955 = property on="time/point, sec" class="DigNum (strict)"() -> ("Value"=w5314:dbl)  [unwired: 2 in, 2 out]
              n3956 = Multiply(x=w5314, y=1000.0) -> (x*y=w5316:dbl)
              n3957 = Subtract(x=w5316, y=w5318) -> (x-y=w5315:dbl)
              n3958 = property on="time delay, ms" class="DigNum (strict)"("Value"=w5315) -> ()  [unwired: 2 in, 2 out]
            }
          }
          n3959 = Or(x=w4338, y="Stop Ramp") -> (x .or. y?=w4339:bool)
        }
        n3960 = stacked-sequence {
          tunnel: w3555 -> [_ _]
          tunnel: w3554 -> [_ w4324]
          frame #0 {
            n3961 = stacked-sequence {
              frame #0 {
                n3962 = local read "sweep"() -> (w4290:T8)
                n3963 = Equal?(x=w4290, y=T17."Radio Selection 7" ("sweep")) -> (x = y?=w4289:bool)
                n3964 = case shown="True" w4289 {
                  frame False {
                  }
                  frame True {
                    n3965 = local read "iPS_addr_sweep"() -> (w4291:refnum<visa-resource-name>)
                    n3966 = call "iPSset.vi"("iPSSetCtrl"=iPSsetCtrl."Hold", "VISA resource name"=w4291) -> ()  [unwired: 6 in, 4 out]
                  }
                }
              }
              frame #1 {
                n3967 = stacked-sequence {
                  frame #0 {
                    n3968 = property on="MFLI1_d0" class="Bool (strict)"() -> ("Value"=w4306:bool)  [unwired: 2 in, 2 out]
                    n3969 = property on="MFLI1_AuxOut0" class="Bool (strict)"() -> ("Value"=w4310:bool)  [unwired: 2 in, 2 out]
                    n3970 = property on="MFLI1_d1" class="Bool (strict)"() -> ("Value"=w4305:bool)  [unwired: 2 in, 2 out]
                    n3971 = property on="MFLI1_d2" class="Bool (strict)"() -> ("Value"=w4304:bool)  [unwired: 2 in, 2 out]
                    n3972 = property on="MFLI1_d3" class="Bool (strict)"() -> ("Value"=w4303:bool)  [unwired: 2 in, 2 out]
                    n3973 = Boolean To (0,1)(Boolean=w4305) -> (0, 1=w4301:i16)
                    n3974 = Boolean To (0,1)(Boolean=w4306) -> (0, 1=w4302:i16)
                    n3975 = Boolean To (0,1)(Boolean=w4310) -> (0, 1=w4307:i16)
                    n3976 = Boolean To (0,1)(Boolean=w4304) -> (0, 1=w4300:i16)
                    n3977 = Boolean To (0,1)(Boolean=w4303) -> (0, 1=w4299:i16)
                    n3978 = Compound Arithmetic op=ADD(w4307, w4302, w4301, w4300, w4299) -> (w4308:i16)
                    n3979 = Greater Than 0?(x=w4308) -> (x > 0?=w4309:bool)
                    n3980 = case shown="True" w4309 {
                      frame False {
                      }
                      frame True {
                        n3981 = property on="HandleOut" class="Clust (strict)"() -> ("Value"=w4311:T1)  [unwired: 2 in, 2 out]
                        n3982 = call <instrlib>:"ziClose.vi"("Handle In"=w4311) -> ()  [unwired: 3 in, 2 out]
                      }
                    }
                  }
                  frame #1 {
                    n3983 = property on="MFLI2_d0" class="Bool (strict)"() -> ("Value"=w4321:bool)  [unwired: 2 in, 2 out]
                    n3984 = property on="MFLI2_d1" class="Bool (strict)"() -> ("Value"=w4317:bool)  [unwired: 2 in, 2 out]
                    n3985 = property on="MFLI2_d2" class="Bool (strict)"() -> ("Value"=w4316:bool)  [unwired: 2 in, 2 out]
                    n3986 = property on="MFLI2_d3" class="Bool (strict)"() -> ("Value"=w4315:bool)  [unwired: 2 in, 2 out]
                    n3987 = Boolean To (0,1)(Boolean=w4316) -> (0, 1=w4312:i16)
                    n3988 = Boolean To (0,1)(Boolean=w4317) -> (0, 1=w4314:i16)
                    n3989 = Boolean To (0,1)(Boolean=w4321) -> (0, 1=w4318:i16)
                    n3990 = Boolean To (0,1)(Boolean=w4315) -> (0, 1=w4313:i16)
                    n3991 = Compound Arithmetic op=ADD(w4318, w4314, w4313, w4312) -> (w4319:i16)
                    n3992 = Greater Than 0?(x=w4319) -> (x > 0?=w4320:bool)
                    n3993 = case shown="True" w4320 {
                      frame False {
                      }
                      frame True {
                        n3994 = property on="HandleOut 2" class="Clust (strict)"() -> ("Value"=w4322:T1)  [unwired: 2 in, 2 out]
                        n3995 = call <instrlib>:"ziClose.vi"("Handle In"=w4322) -> ()  [unwired: 3 in, 2 out]
                      }
                    }
                  }
                }
                n3996 = local read "2636A smua meas v"() -> (w4298:bool)
                n3997 = local read "2636A smub meas v"() -> (w4296:bool)
                n3998 = local read "2636A smub meas i"() -> (w4295:bool)
                n3999 = local read "2636A smua meas i"() -> (w4297:bool)
                n4000 = Compound Arithmetic op=OR(w4298, w4297, w4296, w4295) -> (w4294:bool)
                n4001 = property on="Stop Ramp" class="Bool"("DisabledEnum"=T10."Disabled and Grayed Out" ("Disabled")) -> ()  [unwired: 2 in, 2 out]
                n4002 = case shown="True" w4294 {
                  frame False {
                  }
                  frame True {
                    # "close session on 2636A"
                    n4003 = local read "2614A addr"() -> (w4323:refnum<visa-resource-name>)
                    n4004 = VISA Close(VISA resource name=w4323) -> ()  [unwired: 1 in, 1 out]
                  }
                }
              }
            }
          }
          frame #1 {
            n4005 = property on="Linetrace or Mapping?" class="Bool (strict)"() -> ("Value"=w4325:bool)  [unwired: 2 in, 2 out]
            n4006 = case shown="True" w4325 {
              tunnel: w4324 -> [w4329 w4330]
              frame False {
                w4327 = T10."Enabled" ("Disabled")
                n4007 = Enqueue Element(queue=w4329, element="Idle") -> ()  [unwired: 2 in, 3 out]
                n4008 = property on="sweep" class="RadioBtnsControl (strict)"("DisabledEnum"=w4327) -> ()  [unwired: 2 in, 2 out]
                n4009 = property on="2182A 1 addr" class="DigNum (strict)"("DisabledEnum"=w4327) -> ()  [unwired: 2 in, 2 out]
                n4010 = property on="2182A 2 addr" class="DigNum (strict)"("DisabledEnum"=w4327) -> ()  [unwired: 2 in, 2 out]
                n4011 = property on="2182A 3 addr" class="DigNum (strict)"("DisabledEnum"=w4327) -> ()  [unwired: 2 in, 2 out]
                n4012 = property on="2182A 4 addr" class="DigNum (strict)"("DisabledEnum"=w4327) -> ()  [unwired: 2 in, 2 out]
                n4013 = property on="2400 1 addr" class="DigNum (strict)"("DisabledEnum"=w4327) -> ()  [unwired: 2 in, 2 out]
                n4014 = property on="Sweep Down" class="Bool"("DisabledEnum"=w4327) -> ()  [unwired: 2 in, 2 out]
                n4015 = property on="2400 2 addr" class="DigNum (strict)"("DisabledEnum"=w4327) -> ()  [unwired: 2 in, 2 out]
                n4016 = property on="2400 3 addr" class="DigNum (strict)"("DisabledEnum"=w4327) -> ()  [unwired: 2 in, 2 out]
                n4017 = property on="2614A addr" class="VISAName"("DisabledEnum"=w4327) -> ()  [unwired: 2 in, 2 out]
                n4018 = property on="SR830 1 addr" class="DigNum (strict)"("DisabledEnum"=w4327) -> ()  [unwired: 2 in, 2 out]
                n4019 = property on="SR830 2 addr" class="DigNum (strict)"("DisabledEnum"=w4327) -> ()  [unwired: 2 in, 2 out]
                n4020 = property on="SR830 3 addr" class="DigNum (strict)"("DisabledEnum"=w4327) -> ()  [unwired: 2 in, 2 out]
                n4021 = property on="SR830 4 addr" class="DigNum (strict)"("DisabledEnum"=w4327) -> ()  [unwired: 2 in, 2 out]
                n4022 = property on="Stop Ramp" class="Bool"("DisabledEnum"=T10."Disabled and Grayed Out" ("Disabled")) -> ()  [unwired: 2 in, 2 out]
              }
              frame True {
                n4023 = stacked-sequence {
                  tunnel: w4330 -> [_ w4333]
                  frame #0 {
                    n4024 = property on="Sweep Direction" class="Str"("Value"="Sweep Down" ("Sweep Direction")) -> ()  [unwired: 2 in, 2 out]
                  }
                  frame #1 {
                    n4025 = Enqueue Element(queue=w4333, element="Step to Next Value") -> ()  [unwired: 2 in, 3 out]
                  }
                }
              }
            }
          }
        }
      }
      frame "Step to Next Value" {
        n4026 = property on="Table Index" class="DigNum (strict)"() -> ("Value"=w5335:dbl)  [unwired: 2 in, 2 out]
        n4027 = property on="Step values" class="Tbl (strict)"() -> ("Value"=w5334:string[][])  [unwired: 2 in, 2 out]
        n4028 = Equal?(x=w5335, y=0) -> (x = y?=w5331:bool)
        n4029 = case shown="True" w5331 {
          tunnel: w5335 -> [w5336 w5360]
          tunnel: cluster{"Row":i32, "Column":i32} {"Row"=0, "Column"=0} ("Active Cell:Active Cell") -> [w5340 w5363]
          frame False {
            w5343 = 0 ("Column")
            n4030 = property on="Change Sweep Range" class="Bool (strict)"() -> ("Value"=w5337:bool)  [unwired: 2 in, 2 out]
            n4031 = Decrement(x=w5336) -> (x-1=w5344:dbl)
            n4032 = Bundle By Name(cluster=w5340, "Row"=w5336, "Column"=w5343) -> (w5339:cluster{"Row":i32, "Column":i32})
            n4033 = case shown="True" w5337 {
              tunnel: w5336 -> [_ w5346]
              frame False {
              }
              frame True {
                w5347 = 1 ("Column")
                w5359 = 0 ("Column")
                n4034 = Decrement(x=w5346) -> (x-1=w5358:dbl)
                n4035 = Bundle By Name(cluster=cluster{"Row":i32, "Column":i32} {"Row"=0, "Column"=0} ("Active Cell:Active Cell"), "Row"=w5346, "Column"=w5359) -> (w5356:cluster{"Row":i32, "Column":i32})
                n4036 = Decrement(x=w5346) -> (x-1=w5348:dbl)
                n4037 = Bundle By Name(cluster=w5356, "Row"=w5358, "Column"=w5359) -> (w5355:cluster{"Row":i32, "Column":i32})
                n4038 = Bundle By Name(cluster=cluster{"Row":i32, "Column":i32} {"Row"=0, "Column"=0} ("Active Cell:Active Cell"), "Row"=w5346, "Column"=w5347) -> (w5349:cluster{"Row":i32, "Column":i32})
                n4039 = Bundle By Name(cluster=w5349, "Row"=w5348, "Column"=w5347) -> (w5350:cluster{"Row":i32, "Column":i32})
                n4040 = property on="Down          Up" class="Tbl (strict)"("Active Cell"=w5355, "Cell BG Color"=u32 16711680 ("Active Cell:Cell Background Color")) -> ()  [unwired: 2 in, 2 out]
                n4041 = property on="Down          Up" class="Tbl (strict)"("Active Cell"=w5356, "Cell BG Color"=u32 16776072 ("Active Cell:Cell Background Color")) -> ()  [unwired: 2 in, 2 out]
                n4042 = property on="Down          Up" class="Tbl (strict)"("Active Cell"=w5350, "Cell BG Color"=u32 16711680 ("Active Cell:Cell Background Color")) -> ()  [unwired: 2 in, 2 out]
                n4043 = property on="Down          Up" class="Tbl (strict)"("Active Cell"=w5349, "Cell BG Color"=u32 16776072 ("Active Cell:Cell Background Color")) -> ()  [unwired: 2 in, 2 out]
              }
            }
            n4044 = Bundle By Name(cluster=w5339, "Row"=w5344, "Column"=w5343) -> (w5338:cluster{"Row":i32, "Column":i32})
            n4045 = property on="Step values" class="Tbl (strict)"("Active Cell"=w5339, "Cell BG Color"=u32 16776072 ("Active Cell:Cell Background Color")) -> ()  [unwired: 2 in, 2 out]
            n4046 = property on="Step values" class="Tbl (strict)"("Active Cell"=w5338, "Cell BG Color"=u32 16711680 ("Active Cell:Cell Background Color")) -> ()  [unwired: 2 in, 2 out]
          }
          frame True {
            n4047 = property on="Change Sweep Range" class="Bool (strict)"() -> ("Value"=w5361:bool)  [unwired: 2 in, 2 out]
            n4048 = Bundle By Name(cluster=w5363, "Row"=w5360, "Column"=0) -> (w5362:cluster{"Row":i32, "Column":i32})
            n4049 = case shown="True" w5361 {
              tunnel: w5360 -> [_ w5371]
              frame False {
              }
              frame True {
                w5370 = cluster{"Row":i32, "Column":i32} {"Row"=0, "Column"=0} ("Active Cell:Active Cell")
                n4050 = Bundle By Name(cluster=w5370, "Row"=w5371, "Column"=1) -> (w5367:cluster{"Row":i32, "Column":i32})
                n4051 = Bundle By Name(cluster=w5370, "Row"=w5371, "Column"=0) -> (w5369:cluster{"Row":i32, "Column":i32})
                n4052 = property on="Down          Up" class="Tbl (strict)"("Active Cell"=w5369, "Cell BG Color"=u32 16776072 ("Active Cell:Cell Background Color")) -> ()  [unwired: 2 in, 2 out]
                n4053 = property on="Down          Up" class="Tbl (strict)"("Active Cell"=w5367, "Cell BG Color"=u32 16776072 ("Active Cell:Cell Background Color")) -> ()  [unwired: 2 in, 2 out]
              }
            }
            n4054 = property on="Step values" class="Tbl (strict)"("Active Cell"=w5362, "Cell BG Color"=u32 16776072 ("Active Cell:Cell Background Color")) -> ()  [unwired: 2 in, 2 out]
          }
        }
        n4055 = call <vilib>:"Space Constant.vi"() -> ("String"=w5329:string)
        n4056 = Index Array(array=w5334, index (row)=w5335, index (col)=0 ("disabled index (col)")) -> (element=w5328:string)
        n4057 = call <vilib>:"Search and Replace Pattern.vi"("string"=w5328, "regular expression (\"\")"=w5329, "replace string (\"\")"="" ("replace string (\"\")"), "replace all? (F)"=TRUE) -> ("result string"=w5332:string)  [unwired: 1 in, 1 out]
        n4058 = Equal?(x="", y=w5332) -> (x = y?=w5330:bool)
        n4059 = Fract/Exp String To Number(string=w5332) -> (number=w5333:dbl)  [unwired: 3 in, 1 out]
        n4060 = case shown="False" w5330 {
          tunnel: w5333 -> [w5374 _]
          tunnel: w5322 -> [w5375 w5561]
          frame False {
            # "When step values are not finished"
            n4061 = property on="Current Step Value" class="DigNum (strict)"("Value"=w5374) -> ()  [unwired: 2 in, 2 out]
            n4062 = stacked-sequence {
              tunnel: w5374 -> [w5376 _ _ _]
              tunnel: w5375 -> [_ _ _ w5559]
              frame #0 {
                # "1 = 2400 1\n2 = 2400 2\n\n4 = 2636a smua\n5 = 2636a smub\n6 = do not sweep, just time\n7 = iPS, magnetic field \n8 = iTC, temperature"
                # "set next value in the sweep"
                n4063 = property on="step" class="RadioBtnsControl (strict)"() -> ("Value"=w5377:T5)  [unwired: 2 in, 2 out]
                n4064 = case shown="\"iTC_step\"" w5377 {
                  tunnel: w5376 -> [w5379 w5386 w5392 w5422 _ w5452 w5497 w5524]
                  frame "V2400_1_Step" {
                    # "sweep voltage on 2400 1"
                    n4065 = property on="2400_1_addr_step" class="DigNum (strict)"() -> ("Value"=w5378:u8)  [unwired: 2 in, 2 out]
                    n4066 = Number To Fractional String(number=w5379) -> (F-format string=w5384:string)  [unwired: 3 in]
                    n4067 = Concatenate Strings(":INIT:IMM; :SOUR:VOLT:LEV:IMM:AMPL " ("data"), w5384) -> (w5382:string)
                    n4068 = Number To Decimal String(number=w5378) -> (decimal integer string=w5380:string)  [unwired: 1 in]
                    n4069 = GPIB Write(0:w5380, 1:w5382, 2:i16 1 ("mode (0)")) -> ()  [unwired: 2 in, 2 out]
                  }
                  frame "V2400_2_step" {
                    # "sweep voltage on 2400 2"
                    n4070 = property on="2400_2_addr_step" class="DigNum (strict)"() -> ("Value"=w5385:u8)  [unwired: 2 in, 2 out]
                    n4071 = Number To Fractional String(number=w5386) -> (F-format string=w5391:string)  [unwired: 3 in]
                    n4072 = Concatenate Strings(":INIT:IMM; :SOUR:CURR:LEV:IMM:AMPL " ("data"), w5391) -> (w5389:string)
